vi "Initialize Front Panel.vi"(8 "error in (no error)":errorcluster, 11 "Navigation View in":refnum<class "Navigation View.lvclass">) -> (0 "error out":errorcluster, 3 "Navigation View out":refnum<class "Navigation View.lvclass">)   [LabVIEW 2019, in "Navigation View.lvclass"]
doc: "<License>\nCopyright © 2017 Composed Systems, LLC | All rights reserved\nwww.composed.io\n\nAuthor: Ethan Stern <ethan.stern@composed.io>\n\nThis software is provided \"AS IS\" WITHOUT WARRANTIES, either express or implied, AND IS FOR EDUCATIONAL PURPOSES ONLY.\n</License>"
uses:
  <vilib>/gpm_packages/@cs/Car-wash/Source/Navigation View/Navigation View.lvclass
  <vilib>/gpm_packages/@cs/mva-viewable/Source/IViewable/IViewable/IViewable.lvclass
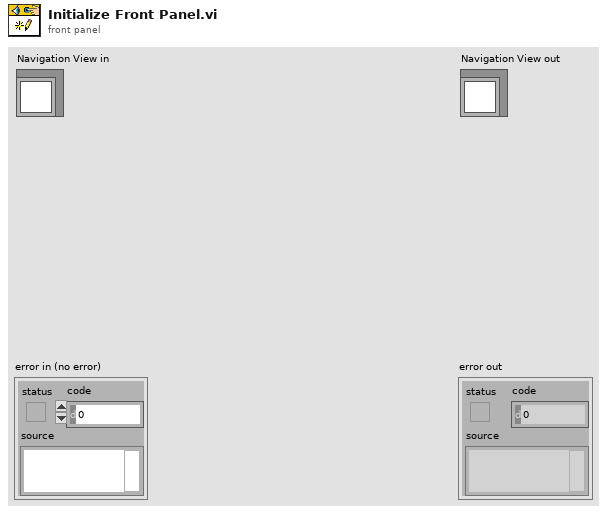
[diagram p1: front panel]
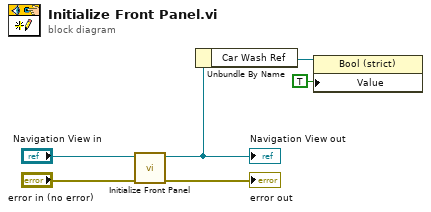
[diagram p0: block diagram]
diagram:
  n1 = call-parent "Initialize Front Panel.vi"("error in (no error)"="error in (no error)", "IViewable in"="Navigation View in") -> ("error out"=→"error out":errorcluster, "IViewable out"=w3:refnum<class "Navigation View.lvclass">)  [unwired: 8 in]
  "Navigation View out" <- w3
  n2 = Unbundle By Name(w3) -> ("Car Wash Ref"=w2:refnum<vi>)
  n3 = property class="Bool (strict)"(reference=w2, "Value"=TRUE) -> ()  [unwired: 1 in, 2 out]
